vi "Save TGA Image (Memory).vi"(8 "error in (no error)":errorcluster, 9 "Compress (T)":bool=TRUE, 10 "Image":T1) -> (0 "error out":errorcluster, 3 "Encoded Image":u8[](array[numeric]))   [LabVIEW 2020, in "G-Image.lvlib"]
doc: "Saves an image in TGA format and returns the encoded image as a byte array.\n\nWhen the <b>Compress</b> input is true, the image is written with run-length encoding (RLE)."
uses:
  G-Image.lvlib
  <vilib>/picture/picture.llb/imagedata.ctl
  Controls/Image Save Format.ctl
  3f50d8b1-806b-44de-96ec-55f047b16f0f.vi
  Private/Result To Error.vi
  Private/Get Image Data.vi
  Private/ARGB To RGBA.vi
  Private/Depth To Number Channels.vi
  Image Processing/To True Color Image.vi
  <vilib>/Utility/error.llb/Error Cluster From Error Code.vi
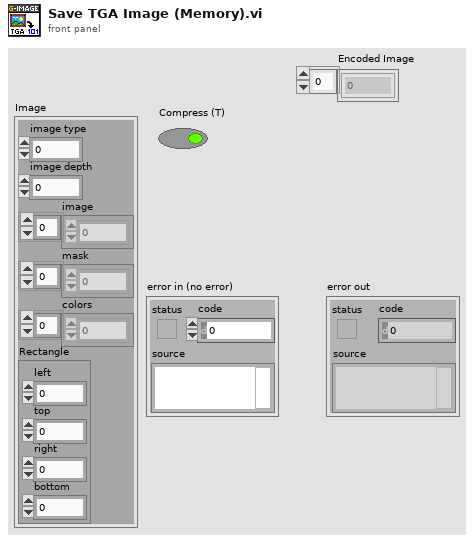
[diagram p1: front panel]
types:
  T1 = typedef "imagedata.ctl" = cluster{"image type":i32, "image depth":i32, "image":u8[], "mask":u8[], "colors":u32[], "Rectangle":cluster{"left":i16, "top":i16, "right":i16, "bottom":i16}}
  T2 = typedef "G-Image.lvlib/Image Save Format.ctl" = enum16{"png", "jpg", "bmp", "gif", "tga", "qoi"}
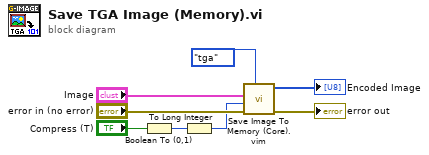
[diagram p0: block diagram]
diagram:
  n1 = Boolean To (0,1)(Boolean="Compress (T)") -> (0, 1=w2:i16)
  n2 = To Long Integer(number=w2) -> (32bit integer=w1:i32)
  n3 = call "Save Image To Memory (Core).vim"("Save Format"=Image_Save_Format."tga", "error in (no error)"="error in (no error)", "Option"=w1, "Image"="Image") -> ("error out"=→"error out":errorcluster, "Encoded Image"=→"Encoded Image":u8[])  [unwired: 6 in]
